vi "ActionVIOnCompile.vi"(8 "error in (no error)":errorcluster, 11 "Device Item Ref in":T2 format="%.0x") -> (0 "error out":errorcluster)   [LabVIEW 2019, in "SLSC-12201 DIO System Explorer.lvlib"]
uses:
  SLSC-12201 DIO System Explorer.lvlib
  <vilib>/NI VeriStand/Custom Device API/Custom Device Item Ref.ctl
  Shared/SLSC Dynamic Channel.ctl
  Shared/SLSC Dynamic Channel Type.ctl
  Shared/Compiled.Settings
  Shared/Constants.vi
  <vilib>/NI VeriStand/Custom Device Tools/Custom Device Utility Library/NI VeriStand - Search for Item by Name.vi
  <vilib>/NI VeriStand/Custom Device API/Get Item Property (I32).vi
  <vilib>/NI VeriStand/Custom Device API/Get Item Property (U32).vi
  <vilib>/NI VeriStand/Custom Device API/Get Item Property (String).vi
  <vilib>/NI VeriStand/Custom Device Tools/Custom Device Utility Library/NI VeriStand - Search for All Items by Name.vi
  <vilib>/NI VeriStand/Custom Device API/Set Item Property (Variant).vi
  <vilib>/NI VeriStand/Custom Device Tools/Custom Device Utility Library/Custom Device Utility Library.lvlib
  <vilib>/NI VeriStand/Custom Device API/Custom Device API.lvlib
  <vilib>/NI/NIVS Inline Async API/_Data Access System Explorer/Data Access System Explorer.lvlib
  Shared/SLSC-12201 DIO Shared.lvlib
panel:
  out "appended array 2":T1(array[cluster]) {"Dev.ProductNumber" format="%.0x"; "Dev.VendorNumber" format="%.0x"}
  out "appended array":T3(array[cluster]) {"VS Refs" format="%.0x"}
  out "SLSC Commands":T4[](array[typedef])
  out "SLSC Set/Write Properties":T4[](array[typedef])
  out "SLSC Get/Read Properties":T4[](array[typedef])
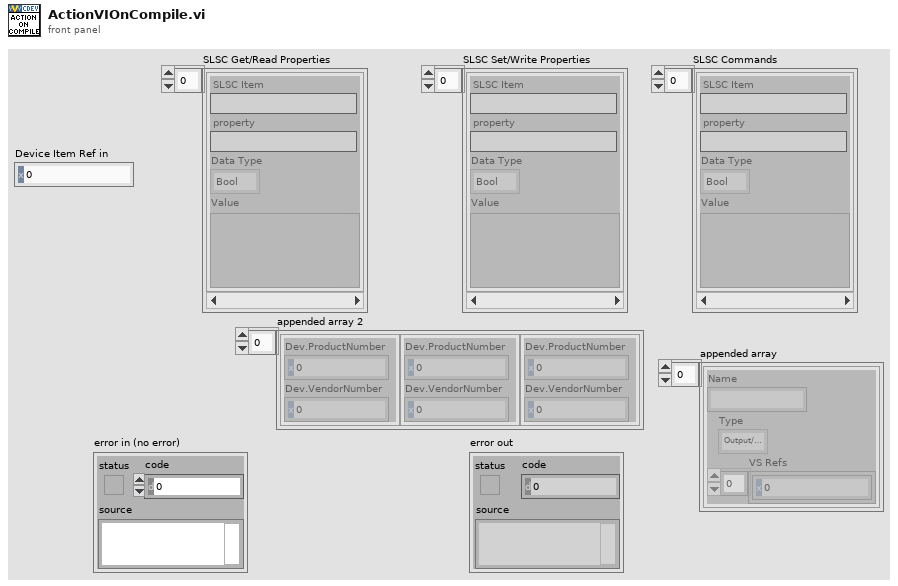
[diagram p1: front panel]
types:
  T1 = cluster{"Dev.ProductNumber":u32, "Dev.VendorNumber":u32}[]
  T2 = typedef "Custom Device API.lvlib/Custom Device Item Ref.ctl" = u64
  T3 = cluster{"Name":string, "Type":enum16{"Output/Write", "Input/Read", "Input/ReadWrite"}, "VS Refs":T2[]}[]
  T4 = typedef "SLSC-12201 DIO Shared.lvlib/SLSC Dynamic Channel.ctl" = cluster{"SLSC Item":string, "property":string, "Data Type":T5, "Value":variant}
  T5 = typedef "SLSC-12201 DIO Shared.lvlib/SLSC Dynamic Channel Type.ctl" = enum16{"Bool", "Double", "I32", "I64", "String", "U32", "U64", "EnumI32"}
  T6 = enum16{"Output/Write", "Input/Read", "Input/ReadWrite"}
  T7 = cluster{"Dev.ProductNumber":u32, "Dev.VendorNumber":u32}
  T8 = typedef "SLSC-12201 DIO Shared.lvlib/Compiled.Settings" = cluster{"Name":string, "SLSC IP -Module Name":string, "Slot #":i32, "Configuration Data":cluster{"Properties":cluster{"Boolean Properties":cluster{"property":refnum<k21>, "Value":bool, "SLSC Item":refnum<k21>}[], "Double Properties":cluster{"property":refnum<k21>, "Double Write":dbl, "SLSC Item":refnum<k21>}[], "I32 Properties":cluster{"property":refnum<k21>, "Int32 Write":i32, "SLSC Item":refnum<k21>}[], "I64 Properties":cluster{"property":refnum<k21>, "Int64 Write":i64, "SLSC Item":refnum<k21>}[], "String Properties":cluster{"property":refnum<k21>, "String Write":string, "SLSC Item":refnum<k21>}[], "U32 Properties":cluster{"property":refnum<k21>, "UInt32 Write":u32, "SLSC Item":refnum<k21>}[], "U64 Properties":cluster{"property":refnum<k21>, "UInt64 Write":u64, "SLSC Item":refnum<k21>}[]}}, "SLSC Set Properties":T4[], "SLSC Get Properties":T4[], "SLSC Commands":T4[], "Username":string, "Password":string, "Support Modules":cluster{"Dev.ProductNumber":u32, "Dev.VendorNumber":u32}[]}
  T9 = cluster{"Name":string, "Type":enum16{"Output/Write", "Input/Read", "Input/ReadWrite"}, "VS Refs":T2[]}
  T10 = typedef "Custom Device API.lvlib/Custom Device Item Info.ctl" = cluster{"Name":string, "Is Channel":bool, "GUID":string, "Is Waveform":bool}
  T11 = cluster{"Properties":cluster{"Boolean Properties":cluster{"property":refnum<k21>, "Value":bool, "SLSC Item":refnum<k21>}[], "Double Properties":cluster{"property":refnum<k21>, "Double Write":dbl, "SLSC Item":refnum<k21>}[], "I32 Properties":cluster{"property":refnum<k21>, "Int32 Write":i32, "SLSC Item":refnum<k21>}[], "I64 Properties":cluster{"property":refnum<k21>, "Int64 Write":i64, "SLSC Item":refnum<k21>}[], "String Properties":cluster{"property":refnum<k21>, "String Write":string, "SLSC Item":refnum<k21>}[], "U32 Properties":cluster{"property":refnum<k21>, "UInt32 Write":u32, "SLSC Item":refnum<k21>}[], "U64 Properties":cluster{"property":refnum<k21>, "UInt64 Write":u64, "SLSC Item":refnum<k21>}[]}}
  T12 = typedef "Custom Device API.lvlib/Custom Device Channel.ctl" = cluster{"Type":T13, "Units":string, "Default Value":dbl, "Faultable":bool, "Scalable":bool}
  T13 = typedef "Custom Device API.lvlib/Custom Device Channel Type.ctl" = enum16{"Input", "Output"}
  T14 = cluster{"Channel Name":string, "SLSC Name":string, "Channel":T12, "Enum Names":string[], "Enum Values":i32[]}[]
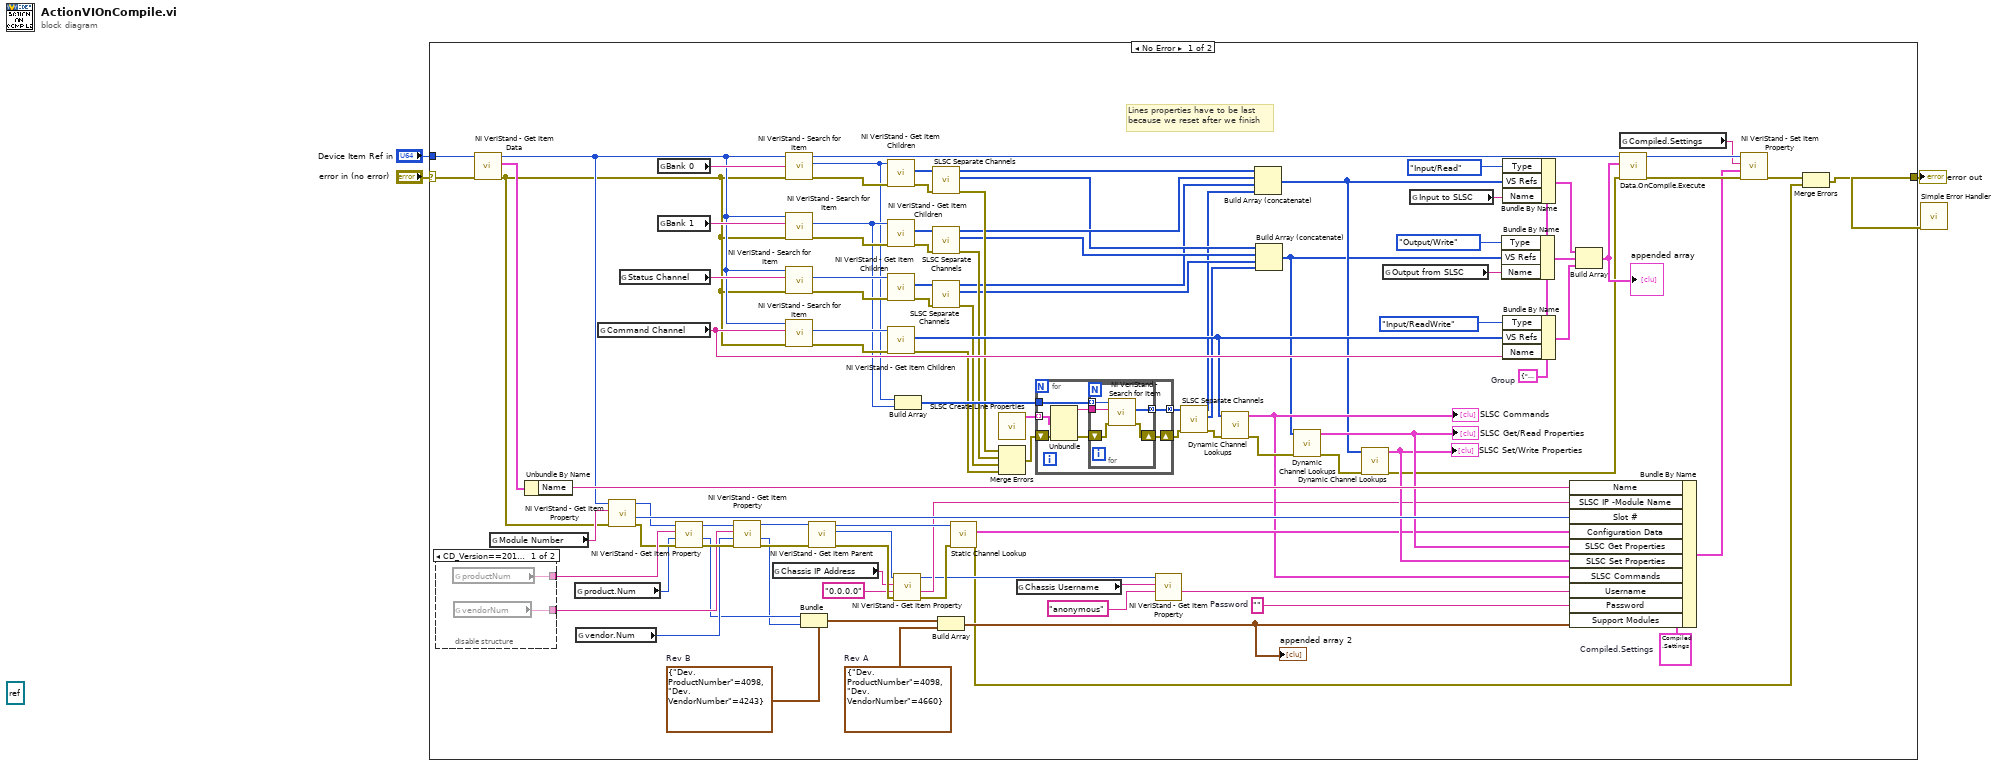
[diagram p0: block diagram]
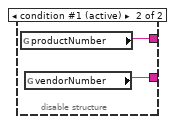
[diagram p2: hidden frame]
diagram:
  (unwired) refnum<k7> refnum ("SHDocVw.IWebBrowser2")
  n1 = case shown="No Error" "error in (no error)" {
    selector: "error in (no error)" -> [w90 w120]
    tunnel: [w88 w120] -> w1
    tunnel: "Device Item Ref in" -> [w91 _]
    frame No Error {
      w6 = T7 {"Dev.ProductNumber"=4098, "Dev.VendorNumber"=4243}  # Rev B
      w12 = T7 {"Dev.ProductNumber"=4098, "Dev.VendorNumber"=4660}  # Rev A
      w64 = ""  # Password
      w81 = T8 {"Name"="", "SLSC IP -Module Name"="", "Slot #"=0, "Configuration Data"={"Properties"={"Boolean Properties"=[], "Double Properties"=[], "I32 Properties"=[], "I64 Properties"=[], "String Properties"=[], "U32 Properties"=[], "U64 Properties"=[]}}, "SLSC Set Properties"=[], "SLSC Get Properties"=[], "SLSC Commands"=[], "Username"="admin", "Password"="", "Support Modules"=[]}  # Compiled.Settings
      w47 = T9 {"Name"="", "Type"=enum."Output/Write", "VS Refs"=[]}  # Group
      # "Lines properties have to be last\nbecause we reset after we finish"
      n2 = disable-structure shown="CD_Version==2015_2016" {
        disable-tunnel: [w106 w108] -> w63
        disable-tunnel: [w105 w107] -> w15
        frame condition #0 {
          n3 = global read "Constants.vi" "productNum"() -> (w106:string)
          n4 = global read "Constants.vi" "vendorNum"() -> (w105:string)
        }
        frame condition #1 (active) {
          n5 = global read "Constants.vi" "productNumber"() -> (w108:string)
          n6 = global read "Constants.vi" "vendorNumber"() -> (w107:string)
        }
      }
      n7 = call <vilib>:"NI VeriStand - Get Item Data.vi"("error in (no error)"=w90, "Item Ref in"=w91) -> ("error out"=w44:errorcluster, "Item Info"=w103:T10, "Item Ref out"=w45:T2)  [unwired: 6 in, 1 out]
      n8 = global read "Constants.vi" "Module Number"() -> (w93:string)
      n9 = Unbundle By Name(w103) -> ("Name"=w102:string)
      n10 = global read "Constants.vi" "product.Num"() -> (w55:i32)
      n11 = global read "Constants.vi" "vendor.Num"() -> (w14:i32)
      n12 = global read "Constants.vi" "Command Channel"() -> (w71:string)
      n13 = call-poly <vilib>:"NI VeriStand - Get Item Property.vi"("error in (no error)"=w44, "Property Name"=w93, "Item Ref in"=w45) -> ("error out"=w61:errorcluster, "Value"=w94:i32, "Item Ref out"=w62:T2)  [unwired: 5 in, 1 out]
      n14 = global read "Constants.vi" "Status Channel"() -> (w76:string)
      n15 = global read "Constants.vi" "Bank 0"() -> (w84:string)
      n16 = global read "Constants.vi" "Bank 1"() -> (w53:string)
      n17 = call-poly <vilib>:"NI VeriStand - Get Item Property.vi"("error in (no error)"=w61, "Default Value"=w55, "Property Name"=w63, "Item Ref in"=w62) -> ("error out"=w16:errorcluster, "Value"=w10:u32, "Item Ref out"=w19:T2)  [unwired: 4 in, 1 out]
      n18 = call-poly <vilib>:"NI VeriStand - Get Item Property.vi"("error in (no error)"=w16, "Default Value"=w14, "Property Name"=w15, "Item Ref in"=w19) -> ("error out"=w17:errorcluster, "Value"=w9:u32, "Item Ref out"=w18:T2)  [unwired: 4 in, 1 out]
      n19 = global read "Constants.vi" "Chassis IP Address"() -> (w92:string)
      n20 = call-poly <vilib>:"NI VeriStand - Search for Item.vi"("error in"=w44, "Item Name"=w84, "Section Ref in"=w45) -> ("error out"=w75:errorcluster, "Item Ref"=w34:T2, "Section Ref out"=w33:T2)  [unwired: 5 in, 1 out]
      n21 = call-poly <vilib>:"NI VeriStand - Search for Item.vi"("error in"=w44, "Item Name"=w53, "Section Ref in"=w45) -> ("error out"=w86:errorcluster, "Item Ref"=w49:T2)  [unwired: 5 in, 2 out]
      n22 = call-poly <vilib>:"NI VeriStand - Search for Item.vi"("error in"=w44, "Item Name"=w76, "Section Ref in"=w45) -> ("error out"=w77:errorcluster, "Item Ref"=w60:T2)  [unwired: 5 in, 2 out]
      n23 = call-poly <vilib>:"NI VeriStand - Search for Item.vi"("error in"=w44, "Item Name"=w71, "Section Ref in"=w45) -> ("error out"=w73:errorcluster, "Item Ref"=w74:T2)  [unwired: 5 in, 2 out]
      n24 = Bundle(cluster=w6, "Dev.ProductNumber"=w10, "Dev.VendorNumber"=w9) -> (w11:T7)
      n25 = call <vilib>:"NI VeriStand - Get Item Parent.vi"("error in (no error)"=w17, "Item Ref in"=w18) -> ("error out"=w96:errorcluster, "Parent Ref"=w95:T2, "Item Ref out"=w78:T2)  [unwired: 6 in, 1 out]
      n26 = call <vilib>:"NI VeriStand - Get Item Children.vi"("error in (no error)"=w75, "Item Ref in"=w34) -> ("error out"=w41:errorcluster, "Child Refs"=w46:T2[])  [unwired: 6 in, 2 out]
      n27 = call <vilib>:"NI VeriStand - Get Item Children.vi"("error in (no error)"=w86, "Item Ref in"=w49) -> ("error out"=w40:errorcluster, "Child Refs"=w51:T2[])  [unwired: 6 in, 2 out]
      n28 = call <vilib>:"NI VeriStand - Get Item Children.vi"("error in (no error)"=w77, "Item Ref in"=w60) -> ("error out"=w39:errorcluster, "Child Refs"=w48:T2[])  [unwired: 6 in, 2 out]
      n29 = call <vilib>:"NI VeriStand - Get Item Children.vi"("error in (no error)"=w73, "Item Ref in"=w74) -> ("error out"=w35:errorcluster, "Child Refs"=w68:T2[])  [unwired: 6 in, 2 out]
      n30 = call-poly <vilib>:"NI VeriStand - Get Item Property.vi"("error in (no error)"=w96, "Default Value"="0.0.0.0", "Property Name"=w92, "Item Ref in"=w95) -> ("error out"=w79:errorcluster, "Value"=w66:string, "Item Ref out"=w57:T2)  [unwired: 4 in, 1 out]
      n31 = Build Array(w34, w49) -> (w50:T2[])
      n32 = call "SLSC Separate Channels.vi"("error in (no error)"=w41, "Item Refs In"=w46) -> ("error out"=w36:errorcluster, "Output Channels"=w30:T2[], "Input Channels"=w32:T2[])  [unwired: 6 in, 1 out]
      n33 = call "SLSC Separate Channels.vi"("error in (no error)"=w40, "Item Refs In"=w51) -> ("error out"=w37:errorcluster, "Output Channels"=w29:T2[], "Input Channels"=w31:T2[])  [unwired: 6 in, 1 out]
      n34 = call "SLSC Separate Channels.vi"("error in (no error)"=w39, "Item Refs In"=w48) -> ("error out"=w38:errorcluster, "Output Channels"=w28:T2[], "Input Channels"=w8:T2[])  [unwired: 6 in, 1 out]
      n35 = Build Array(w11, w12) -> (w13:T1)
      "appended array 2" <- w13
      n36 = call "Static Channel Lookup.vi"("error in (no error)"=w79, "Device Item Ref in"=w78) -> ("error out"=w4:errorcluster, "Configuration Data"=w80:T11)  [unwired: 7 in, 1 out]
      n37 = call "SLSC Create Line Properties.vi"() -> ("Outgoing configuration"=w52:T14)  [unwired: 11 in]
      n38 = Merge Errors(w36, w37, w38, w35) -> (w43:errorcluster)
      n39 = global read "Constants.vi" "Chassis Username"() -> (w58:string)
      n40 = for {
        tunnel: w52 -> [w114] mode=indexing
        tunnel: [w112] -> w25 mode=concatenating
        shift-right: [w110] -> w21
        shift-left: w43 -> [w111]
        tunnel: w50 -> [w109]
        n41 = Unbundle(w114) -> ("Channel Name"=w113:string)  [unwired: 4 out]
        n42 = for {
          tunnel: w113 -> [w119]
          tunnel: [w118] -> w112 mode=concatenating
          tunnel: w109 -> [w115] mode=indexing
          shift-right: [w116] -> w110
          shift-left: w111 -> [w117]
          n43 = call-poly <vilib>:"NI VeriStand - Search for Item.vi"("error in"=w117, "Item Name"=w119, "Section Ref in"=w115) -> ("error out"=w116:errorcluster, "Item Refs"=w118:T2[])  [unwired: 5 in, 2 out]
        }
      }
      n44 = call-poly <vilib>:"NI VeriStand - Get Item Property.vi"("Default Value"="anonymous", "Property Name"=w58, "Item Ref in"=w57) -> ("Value"=w56:string)  [unwired: 5 in, 3 out]
      n45 = call "SLSC Separate Channels.vi"("error in (no error)"=w21, "Item Refs In"=w25) -> ("error out"=w20:errorcluster, "Output Channels"=w24:T2[], "Input Channels"=w7:T2[])  [unwired: 6 in, 1 out]
      n46 = call "Dynamic Channel Lookups.vi"("error in (no error)"=w20, "Child Refs"=w68) -> ("error out"=w69:errorcluster, "SLSC Dynamic Inputs"=w67:T4[])  [unwired: 8 in]
      "SLSC Commands" <- w67
      n47 = Build Array (concatenate)(w32, w31, w8, w7) -> (w23:T2[])
      n48 = Build Array (concatenate)(w30, w29, w28, w24) -> (w22:T2[])
      n49 = call "Dynamic Channel Lookups.vi"("error in (no error)"=w69, "Child Refs"=w22) -> ("error out"=w85:errorcluster, "SLSC Dynamic Inputs"=w87:T4[])  [unwired: 8 in]
      "SLSC Get/Read Properties" <- w87
      n50 = call "Dynamic Channel Lookups.vi"("error in (no error)"=w85, "Child Refs"=w23) -> ("error out"=w42:errorcluster, "SLSC Dynamic Inputs"=w82:T4[])  [unwired: 8 in]
      "SLSC Set/Write Properties" <- w82
      n51 = global read "Constants.vi" "Output from SLSC"() -> (w83:string)
      n52 = global read "Constants.vi" "Input to SLSC"() -> (w54:string)
      n53 = Bundle By Name(cluster=w47, "Type"=T6."Output/Write", "VS Refs"=w22, "Name"=w83) -> (w26:T9)
      n54 = Bundle By Name(cluster=w47, "Type"=T6."Input/Read", "VS Refs"=w23, "Name"=w54) -> (w27:T9)
      n55 = Bundle By Name(cluster=w47, "Type"=T6."Input/ReadWrite", "VS Refs"=w68, "Name"=w71) -> (w70:T9)
      n56 = Bundle By Name(cluster=w81, "Name"=w102, "SLSC IP -Module Name"=w66, "Slot #"=w94, "Configuration Data"=w80, "SLSC Get Properties"=w87, "SLSC Set Properties"=w82, "SLSC Commands"=w67, "Username"=w56, "Password"=w64, "Support Modules"=w13) -> (w5:T8)
      n57 = Build Array(w27, w26, w70) -> (w100:T3)
      "appended array" <- w100
      n58 = global read "Constants.vi" "Compiled.Settings"() -> (w89:string)
      n59 = call <vilib>:"Data.OnCompile.Execute.vi"("error in"=w42, "VS Ref Groups"=w100, "Custom Device Ref"=w33) -> ("error out"=w98:errorcluster, "Custom Device Ref"=w97:T2)  [unwired: 7 in]
      n60 = call-poly <vilib>:"NI VeriStand - Set Item Property.vi"("error in (no error)"=w98, "Value"=w5, "Property Name"=w89, "Item Ref in"=w97) -> ("error out"=w104:errorcluster)  [unwired: 5 in, 2 out]
      n61 = Merge Errors(w104, w4) -> (w88:errorcluster)
    }
    frame Error {
    }
  }
  "error out" <- w1
  n62 = call <vilib>:"Simple Error Handler.vi"("error in (no error)"=w1) -> ()  [unwired: 4 in, 5 out]
